vi "SetMeasurementParameters.vi"(8 "error in (no error)":errorcluster) -> (0 "error out":errorcluster)   [LabVIEW 2015, in "ESLSCDLL.lvlib"]
uses:
  ESLSCDLL.lvlib
  Globals.vi
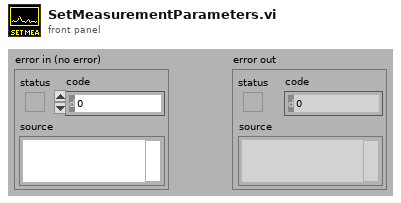
[diagram p1: front panel]
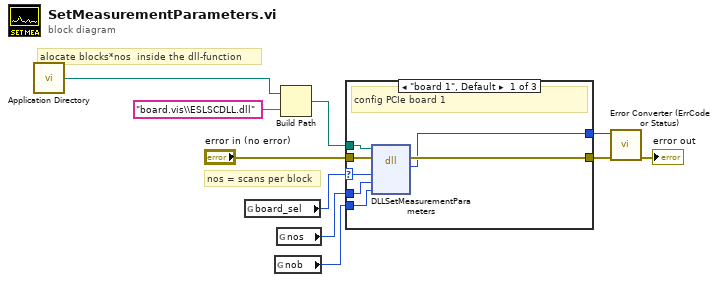
[diagram p0: block diagram]
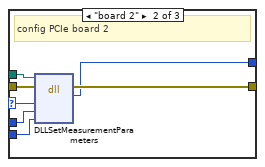
[diagram p2: hidden frame]
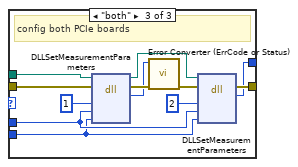
[diagram p3: hidden frame]
diagram:
  # "alocate blocks*nos  inside the dll-function"
  # "nos = scans per block"
  n1 = call <vilib>:"Application Directory.vi"() -> ("Application Directory"=w3:path)
  n2 = global read "Globals.vi" "board_sel"() -> (w6:enum32{"0", "board 1", "board 2", "both"})
  n3 = global read "Globals.vi" "nob"() -> (w4:u32)
  n4 = global read "Globals.vi" "nos"() -> (w5:u32)
  n5 = Build Path(base path=w3, name or relative path="board.vis\\ESLSCDLL.dll") -> (appended path=w1:path)
  n6 = case shown="\"board 1\", Default" w6 {
    selector: w6 -> [w17 w22 _]
    tunnel: w4 -> [w16 w24 w33]
    tunnel: w5 -> [w15 w23 w34]
    tunnel: "error in (no error)" -> [w14 w21 w32]
    tunnel: [w13 w20 w28] -> w8
    tunnel: [w12 w19 w27] -> w7
    tunnel: w1 -> [w11 w18 w26]
    frame "board 1", Default {
      # "config PCIe board 1"
      n7 = dll-call lib="C:/ENTW/PCIE/LV64/board.vis/ESLSCDLL.dll" fn="DLLSetMeasurementParameters" ("lwlscdll.dll:DLLReadFFLoop")(path in=w11, error in=w14, "drv"=w17, "nos"=w15, "nob"=w16) -> (error out=w13:errorcluster, "es_status_codes"=w12:i32)  [unwired: 4 in, 1 out]
    }
    frame "board 2" {
      # "config PCIe board 2"
      n8 = dll-call lib="C:/ENTW/PCIE/LV64/board.vis/ESLSCDLL.dll" fn="DLLSetMeasurementParameters" ("lwlscdll.dll:DLLReadFFLoop")(path in=w18, error in=w21, "drv"=w22, "nos"=w23, "nob"=w24) -> (error out=w20:errorcluster, "es_status_codes"=w19:i32)  [unwired: 4 in, 1 out]
    }
    frame "both" {
      # "config both PCIe boards"
      n9 = dll-call lib="C:/ENTW/PCIE/LV64/board.vis/ESLSCDLL.dll" fn="DLLSetMeasurementParameters" ("lwlscdll.dll:DLLReadFFLoop")(path in=w26, error in=w32, "drv"=u32 1, "nos"=w34, "nob"=w33) -> (path out=w25:path, error out=w31:errorcluster, "es_status_codes"=w30:i32)  [unwired: 4 in]
      n10 = call "Error Converter (ErrCode or Status).vi"("error in (no error)"=w31, "error code"=w30) -> ("error out"=w29:errorcluster)  [unwired: 9 in]
      n11 = dll-call lib="C:/ENTW/PCIE/LV64/board.vis/ESLSCDLL.dll" fn="DLLSetMeasurementParameters" ("lwlscdll.dll:DLLReadFFLoop")(path in=w25, error in=w29, "drv"=u32 2, "nos"=w34, "nob"=w33) -> (error out=w28:errorcluster, "es_status_codes"=w27:i32)  [unwired: 4 in, 1 out]
    }
  }
  n12 = call "Error Converter (ErrCode or Status).vi"("error in (no error)"=w8, "error code"=w7) -> ("error out"=→"error out":errorcluster)  [unwired: 9 in]
